vi "Create HTML.vi"(8 "error in (no error)":errorcluster, 11 "Web FP In":refnum<class "Web Front Panel.lvclass">) -> (0 "error out":errorcluster, 1 "HTML":string, 2 "js":string, 3 "Web FP Out":refnum<class "Web Front Panel.lvclass">, 5 "Name":string)   [LabVIEW 2017, in "Front Panel Publisher.lvlib" / "Web Front Panel.lvclass"]
uses:
  Web Front Panel.lvclass
  Controls/HTML Template Fill.ctl
  Controls/JS Template Fill.ctl
  Web Front Panel.lvclass/Web Front Panel.ctl
  <userlib>/_OpenG.lib/array/array.llb/Remove Duplicates from 1D Array (String)__ogtk.vi
  Front Panel Objects/Object_class/Object.lvclass
  Front Panel Manager_class/Front Panel Manager.lvclass
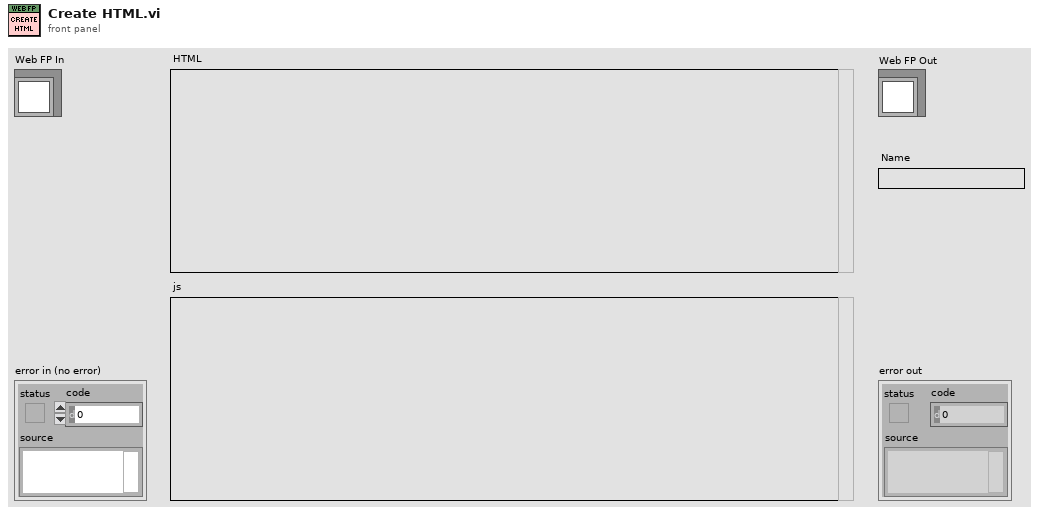
[diagram p1: front panel]
types:
  T1 = typedef "Front Panel Publisher.lvlib/Web Front Panel.lvclass/JS Template Fill.ctl" = cluster{"Page Name":string, "js varibles":string, "Code for controls":string, "Code for indicators":string, "Refresh rate (ms)":i32}
  T2 = typedef "Front Panel Publisher.lvlib/Web Front Panel.lvclass/HTML Template Fill.ctl" = cluster{"Page Name":string, "Script dependencies":string, "Body width (px)":i32, "Body height (px)":i32, "Background Colour":u32, "HTML elements":string}
  T3 = typedef "Front Panel Publisher.lvlib/Web Front Panel.lvclass/Object Attributes.ctl" = cluster{"VI Identifier":string, "VI Reference":refnum<vi>, "Controls":refnum<class "Object.lvclass">[], "Indicators":refnum<class "Object.lvclass">[], "Decorations":refnum<class "Object.lvclass">[], "VR With Previous Get":refnum<data-value>, "VR With Ring Images":refnum<data-value>}
  T4 = typedef "Front Panel Publisher.lvlib/Web Front Panel.lvclass/High Level Config Settings.ctl" = cluster{"Default Refresh Rate (ms)":i32, "Show Border":bool, "Periodic Decoration Data":bool, "Synchronous Requests":bool, "Reduce Sent Data":bool, "Recommended Control Settings":bool}
  T5 = typedef "LVRectTypeDef.ctl" = cluster{"Left":i16, "Top":i16, "Right":i16, "Bottom":i16}
  T6 = typedef "Front Panel Publisher.lvlib/Front Panel Manager.lvclass/Websocket Info.ctl" = cluster{"Hostname":string, "Port":u16}
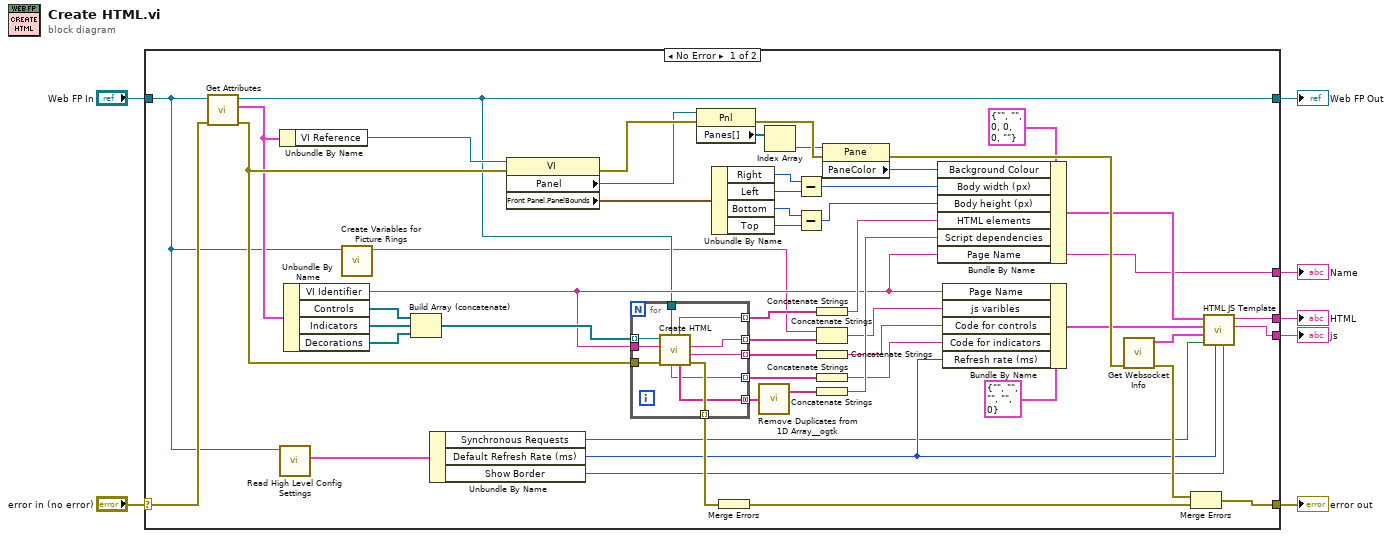
[diagram p0: block diagram]
diagram:
  n1 = case shown="No Error" "error in (no error)" {
    selector: "error in (no error)" -> [w59 w71]
    tunnel: [w54 w71] -> w6
    tunnel: [w15 w70] -> w4
    tunnel: "Web FP In" -> [w12 w70]
    tunnel: [w33 _] -> w3
    tunnel: [w17 _] -> w2
    tunnel: [w19 _] -> w1
    frame No Error {
      n2 = call "Get Attributes.vi"("error in (no error)"=w59, "Web FP In"=w12) -> ("error out"=w57:errorcluster, "Data"=w37:T3, "Web FP Out"=w15:refnum<class "Web Front Panel.lvclass">)  [unwired: 6 in, 1 out]
      n3 = Unbundle By Name(w37) -> ("VI Reference"=w41:refnum<vi>)
      n4 = call "Read High Level Config Settings.vi"("Web FP In"=w12) -> ("High Level Config Settings"=w11:T4)  [unwired: 8 in, 2 out]
      n5 = Unbundle By Name(w37) -> ("VI Identifier"=w19:string, "Controls"=w36:refnum<class "Object.lvclass">[], "Indicators"=w35:refnum<class "Object.lvclass">[], "Decorations"=w13:refnum<class "Object.lvclass">[])
      n6 = call "Create Variables for Picture Rings.vi"("Web FP In"=w12) -> ("Variables String"=w14:string)  [unwired: 9 in, 1 out]
      n7 = Build Array (concatenate)(w36, w35, w13) -> (w38:refnum<class "Object.lvclass">[])
      n8 = Unbundle By Name(w11) -> ("Synchronous Requests"=w8:bool, "Default Refresh Rate (ms)"=w9:i32, "Show Border"=w10:bool)
      n9 = property class="VI"(reference=w41, error in=w57) -> (error out=w56:errorcluster, "Panel"=w26:refnum<vi>, "Front Panel.PanelBounds"=w46:T5)  [unwired: 1 out]
      n10 = for {
        tunnel: w38 -> [w67] mode=indexing
        tunnel: [w66] -> w51 mode=indexing
        tunnel: [w65] -> w50 mode=indexing
        tunnel: [w64] -> w49 mode=indexing
        tunnel: [w63] -> w48 mode=concatenating
        tunnel: w57 -> [w69]
        tunnel: [w68] -> w40 mode=indexing
        tunnel: [w62] -> w39 mode=indexing
        tunnel: w19 -> [w61]
        tunnel: w15 -> [w60]
        n11 = call-dynamic "Create HTML.vi"("FP Reference"=w60, "error in (no error)"=w69, "VI Identifier"=w61, "Object In"=w67) -> ("error out"=w68:errorcluster, "js code for controls"=w64:string, "js variables"=w65:string, "script dependencies"=w63:string[], "HTML"=w66:string, "js code for indicators"=w62:string)  [unwired: 1 in, 1 out]
      }
      n12 = property class="Pnl"(reference=w26, error in=w56) -> (error out=w55:errorcluster, "Panes[]"=w28:refnum<vi>[])  [unwired: 1 out]
      n13 = Unbundle By Name(w46) -> ("Right"=w45:i16, "Left"=w44:i16, "Bottom"=w43:i16, "Top"=w42:i16)
      n14 = Merge Errors(w40) -> (w58:errorcluster)
      n15 = call-poly <userlib>:"Remove Duplicates from 1D Array__ogtk.vi"("Input Array"=w48) -> ("Output Array"=w47:string[])  [unwired: 1 out]
      n16 = Index Array(array=w28) -> (element=w27:refnum<vi>)  [unwired: 1 in]
      n17 = Subtract(x=w45, y=w44) -> (x-y=w32:i16)
      n18 = Subtract(x=w43, y=w42) -> (x-y=w31:i16)
      n19 = Concatenate Strings(w51) -> (w30:string)
      n20 = Concatenate Strings(w14, w50) -> (w22:string)
      n21 = Concatenate Strings(w49) -> (w21:string)
      n22 = Concatenate Strings(w39) -> (w20:string)
      n23 = Concatenate Strings(w47) -> (w29:string)
      n24 = property class="Pane"(reference=w27, error in=w55) -> (error out=w53:errorcluster, "PaneColor"=w25:u32)  [unwired: 1 out]
      n25 = Bundle By Name(cluster=T2 {"Page Name"="", "Script dependencies"="", "Body width (px)"=0, "Body height (px)"=0, "Background Colour"=0, "HTML elements"=""} ("HTML"), "Background Colour"=w25, "Body width (px)"=w32, "Body height (px)"=w31, "HTML elements"=w30, "Script dependencies"=w29, "Page Name"=w19) -> (w24:T2)
      n26 = Bundle By Name(cluster=T1 {"Page Name"="", "js varibles"="", "Code for controls"="", "Code for indicators"="", "Refresh rate (ms)"=0} ("js"), "Page Name"=w19, "js varibles"=w22, "Code for controls"=w21, "Code for indicators"=w20, "Refresh rate (ms)"=w9) -> (w18:T1)
      n27 = call "Get Websocket Info.vi"("error in (no error)"=w53) -> ("error out"=w52:errorcluster, "Connection Info"=w16:T6)  [unwired: 9 in]
      n28 = Merge Errors(w52, w58) -> (w54:errorcluster)
      n29 = call "HTML JS Template.vi"("Show Border"=w10, "Refresh rate (250ms)"=w9, "Synchronous Requests"=w8, "Websocket Info"=w16, "js"=w18, "HTML"=w24) -> ("js out"=w17:string, "HTML out"=w33:string)  [unwired: 4 in]
    }
    frame Error {
    }
  }
  "error out" <- w6
  "Web FP Out" <- w4
  "HTML" <- w3
  "js" <- w2
  "Name" <- w1
